vi "SimpleRTFIFO.vi"() -> ()   [LabVIEW 2015]
uses:
  <vilib>/real-time/rtfifo.llb/RTFIFOCreate I32.vi
  <vilib>/real-time/rtfifo.llb/RTFIFOWrite I32.vi
  <vilib>/real-time/rtfifo.llb/RTFIFORead I32.vi
  <vilib>/real-time/rtfifo.llb/RTFIFODelete I32.vi
  <vilib>/real-time/NI_Real-Time Libraries.lvlib
panel:
  out "overwrite (third write)":bool
  out "overwrite (first write)":bool
  out "overwrite (second write)":bool
  out "FIFO 3 first element out":i32
  out "empty (second read)":bool
  out "empty (first read)":bool
  out "FIFO 2 second element out":i32
  out "FIFO 2 first element out":i32
  out "FIFO1 first element out":i32
  # "These are not actual use cases, but are only meant to serve as a tutorial for learning the basics of RTFIFOs.  FIFO stands for \nFirst In First Out, and is similar to a queue. RTFIFO's are meant to be used for communicating data between a time critical \nthread and lower priority threads without harming determinism (as in the case of using queues, notifiers, and global variables)."
  # "Output for Example 1"
  # "Example 1.  This is a simple example of creating a FIFO, performing\none write and one read, and then deleting the FIFO."
  # "Output for Example 2"
  # "Example 2.  This example builds on example 1, but demonstrates that\nthe RTFIFORead.vi will return the input value if the FIFO is empty. \nOnly one element is written, but there are two reads.  Since the FIFO\nis empty for the second read, the input element is returned."
  # "Example 3.  This example builds on example 1, but demonstrates that\nthe RTFIFOWrite.vi will overwrite the oldest element in the FIFO if the\nFIFO is full.  This example uses a FIFO size of 2.  Even though 100 \nwas written to the FIFO first, after writing a 200, then a 300, since the \nFIFO is only two elements long, the the first element is removed from \nthe FIFO, and only the second and third elements remain."
  # "Output for Example 3"
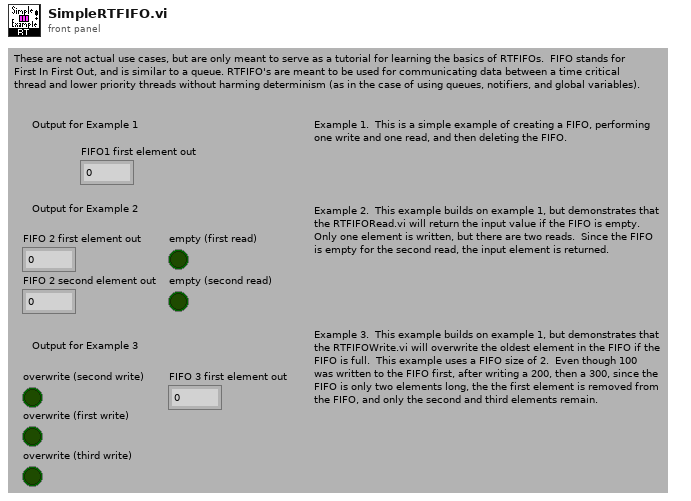
[diagram p1: front panel]
types:
  T1 = typedef "NI_Real-Time Libraries.lvlib/RTFIFORefnum I32.ctl" = cluster{"index":u32, "id":u32, "type":i32, "size":u32}
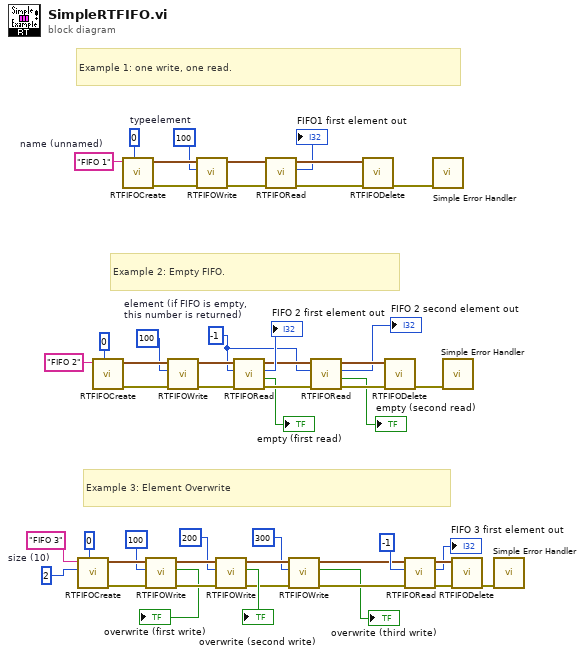
[diagram p0: block diagram]
diagram:
  w7 = u32 2  # size (10)
  w23 = -1  # element (if FIFO is empty,  this number is returned)
  w41 = 100  # element
  w49 = "FIFO 1"  # name (unnamed)
  w50 = 0  # type
  # "Example 3: Element Overwrite"
  # "Example 2: Empty FIFO."
  # "Example 1: one write, one read."
  n1 = call-poly <vilib>:"RTFIFOCreate.vi"("type"=0, "size (10)"=w7, "name (unnamed)"="FIFO 3") -> ("error out"=w20:errorcluster, "rt fifo"=w18:T1)  [unwired: 2 in, 5 out]
  n2 = call-poly <vilib>:"RTFIFOCreate.vi"("type"=0, "name (unnamed)"="FIFO 2") -> ("error out"=w37:errorcluster, "rt fifo"=w35:T1)  [unwired: 3 in, 5 out]
  n3 = call-poly <vilib>:"RTFIFOCreate.vi"("type"=w50, "name (unnamed)"=w49) -> ("error out"=w48:errorcluster, "rt fifo"=w45:T1)  [unwired: 3 in, 5 out]
  n4 = call-poly <vilib>:"RTFIFOWrite.vi"("error in (no error)"=w20, "element"=100, "rt fifo"=w18) -> ("error out"=w19:errorcluster, "overwrite"=→"overwrite (first write)":bool, "rt fifo out"=w17:T1)  [unwired: 6 out]
  n5 = call-poly <vilib>:"RTFIFOWrite.vi"("error in (no error)"=w37, "element"=100, "rt fifo"=w35) -> ("error out"=w36:errorcluster, "rt fifo out"=w34:T1)  [unwired: 7 out]
  n6 = call-poly <vilib>:"RTFIFOWrite.vi"("error in (no error)"=w48, "element"=w41, "rt fifo"=w45) -> ("error out"=w47:errorcluster, "rt fifo out"=w44:T1)  [unwired: 7 out]
  n7 = call-poly <vilib>:"RTFIFOWrite.vi"("error in (no error)"=w19, "element"=200, "rt fifo"=w17) -> ("error out"=w5:errorcluster, "overwrite"=→"overwrite (second write)":bool, "rt fifo out"=w6:T1)  [unwired: 6 out]
  n8 = call-poly <vilib>:"RTFIFORead.vi"("error in (no error)"=w36, "element"=w23, "rt fifo"=w34) -> ("error out"=w30:errorcluster, "empty"=→"empty (first read)":bool, "element out"=→"FIFO 2 first element out":i32, "rt fifo out"=w28:T1)  [unwired: 5 out]
  n9 = call-poly <vilib>:"RTFIFORead.vi"("error in (no error)"=w47, "rt fifo"=w44) -> ("error out"=w46:errorcluster, "element out"=→"FIFO1 first element out":i32, "rt fifo out"=w43:T1)  [unwired: 1 in, 6 out]
  n10 = call-poly <vilib>:"RTFIFOWrite.vi"("error in (no error)"=w5, "element"=300, "rt fifo"=w6) -> ("error out"=w4:errorcluster, "overwrite"=→"overwrite (third write)":bool, "rt fifo out"=w3:T1)  [unwired: 6 out]
  n11 = call-poly <vilib>:"RTFIFORead.vi"("error in (no error)"=w30, "element"=w23, "rt fifo"=w28) -> ("error out"=w29:errorcluster, "empty"=→"empty (second read)":bool, "element out"=→"FIFO 2 second element out":i32, "rt fifo out"=w27:T1)  [unwired: 5 out]
  n12 = call-poly <vilib>:"RTFIFODelete.vi"("error in (no error)"=w46, "rt fifo"=w43) -> ("error out"=w42:errorcluster)  [unwired: 9 out]
  n13 = call-poly <vilib>:"RTFIFODelete.vi"("error in (no error)"=w29, "rt fifo"=w27) -> ("error out"=w33:errorcluster)  [unwired: 9 out]
  n14 = call-poly <vilib>:"RTFIFORead.vi"("error in (no error)"=w4, "element"=-1, "rt fifo"=w3) -> ("error out"=w14:errorcluster, "element out"=→"FIFO 3 first element out":i32, "rt fifo out"=w13:T1)  [unwired: 6 out]
  n15 = call <vilib>:"Simple Error Handler.vi"("error in (no error)"=w42) -> ()  [unwired: 1 in, 8 out]
  n16 = call <vilib>:"Simple Error Handler.vi"("error in (no error)"=w33) -> ()  [unwired: 1 in, 8 out]
  n17 = call-poly <vilib>:"RTFIFODelete.vi"("error in (no error)"=w14, "rt fifo"=w13) -> ("error out"=w16:errorcluster)  [unwired: 9 out]
  n18 = call <vilib>:"Simple Error Handler.vi"("error in (no error)"=w16) -> ()  [unwired: 1 in, 8 out]
